vi "fx3u以太网通讯.vi"() -> ()   [LabVIEW 2017]
uses:
  C:/Users/Administrator/Desktop/LV2014_HslCommunication/LV2014_HslCommunication/HslCommunication.dll
  LV2014_HslCommunication/LV2014_HslCommunication/HslCommunication.dll
panel:
  out "Content 2":u32[](array[numeric])
  in  "布尔":bool
  out "IsSuccess 2":bool
  out "Content":i16
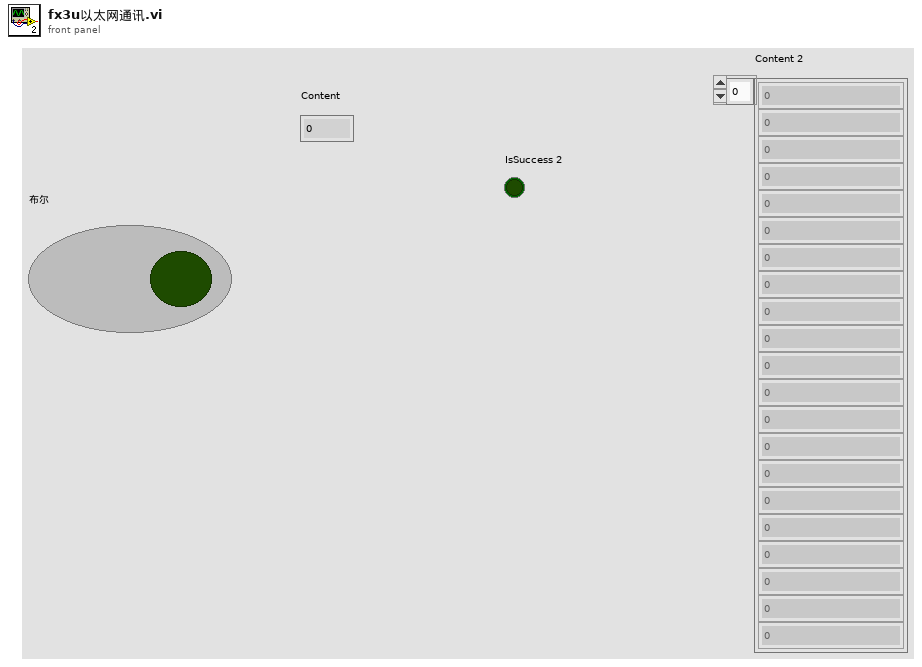
[diagram p1: front panel]
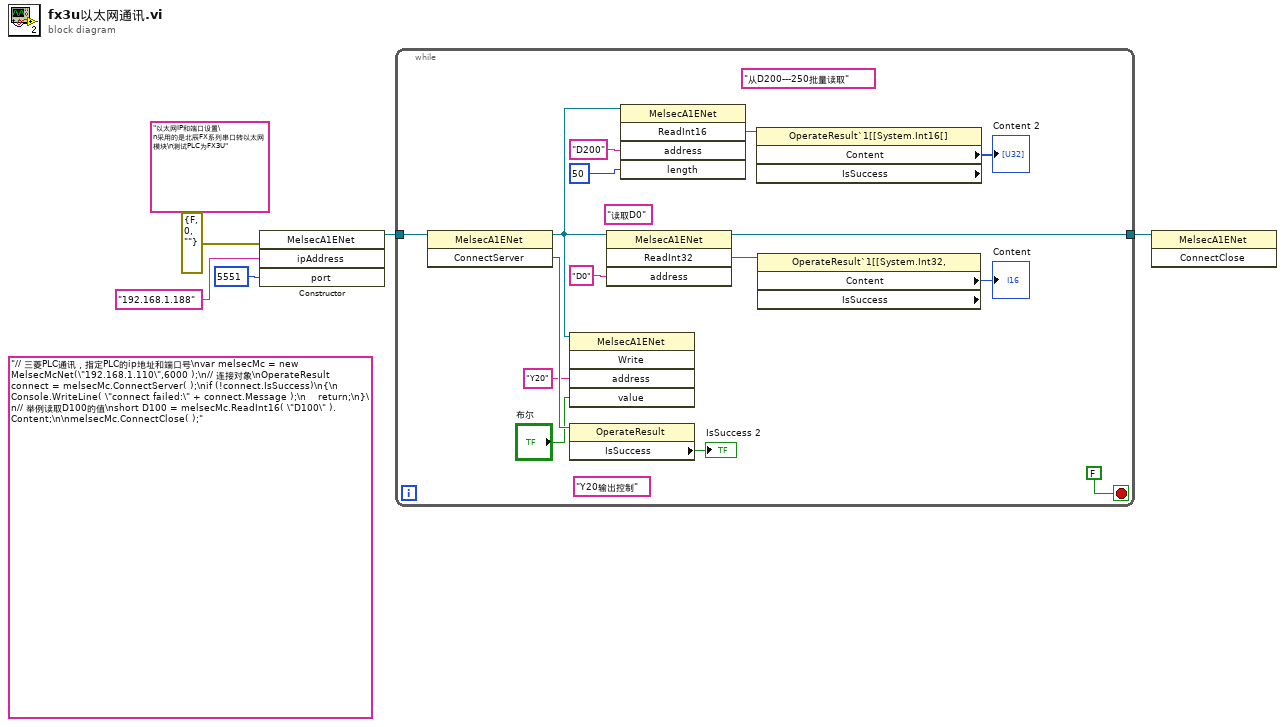
[diagram p0: block diagram]
diagram:
  (unwired) "以太网IP和端口设置\n采用的是北辰FX系列串口转以太网模块\n测试PLC为FX3U"
  (unwired) "// 三菱PLC通讯，指定PLC的ip地址和端口号\nvar melsecMc = new MelsecMcNet(\"192.168.1.110\",6000 );\n// 连接对象\nOperateResult connect = melsecMc.ConnectServer( );\nif (!connect.IsSuccess)\n{\n    Console.WriteLine( \"connect failed:\" + connect.Message );\n    return;\n}\n// 举例读取D100的值\nshort D100 = melsecMc.ReadInt16( \"D100\" ).Content;\n\nmelsecMc.ConnectClose( );"
  n1 = constructor class="MelsecA1ENet"(error in=errorcluster {"status"=FALSE, "code"=0, "source"=""} ("错误输入（无错误）"), "ipAddress"="192.168.1.188", "port"=5551) -> (reference out=w3:refnum<k24>)  [unwired: 2 in, 4 out]
  n2 = while {
    tunnel: [w16] -> w4
    tunnel: w3 -> [w14]
    stop <- FALSE stop-if-true
    (unwired) "读取D0"
    (unwired) "从D200---250批量读取"
    (unwired) "Y20输出控制"
    n3 = invoke class="MelsecA1ENet" method="ConnectServer"(reference=w14) -> (reference out=w10:refnum<k24>, "ConnectServer"=w13:refnum<k24>)  [unwired: 2 in, 1 out]
    n4 = invoke class="MelsecA1ENet" method="Write"(reference=w10, "address"="Y20", "value"="布尔") -> ()  [unwired: 2 in, 5 out]
    n5 = property class="OperateResult"(reference=w13) -> ("IsSuccess"=→"IsSuccess 2":bool)  [unwired: 1 in, 2 out]
    n6 = invoke class="MelsecA1ENet" method="ReadInt32"(reference=w10, "address"="D0") -> (reference out=w16:refnum<k24>, "ReadInt32"=w19:refnum<k24>)  [unwired: 2 in, 2 out]
    n7 = invoke class="MelsecA1ENet" method="ReadInt16"(reference=w10, "address"="D200", "length"=u16 50) -> ("ReadInt16"=w8:refnum<k24>)  [unwired: 2 in, 4 out]
    n8 = property class="OperateResult`1[[System.Int16[]" props=["Content", "IsSuccess"](reference=w8) -> ("Content"=→"Content 2":i16[])  [unwired: 1 in, 3 out]
    n9 = property class="OperateResult`1[[System.Int32, " props=["Content", "IsSuccess"](reference=w19) -> ("Content"=→"Content":i32)  [unwired: 1 in, 3 out]
  }
  n10 = invoke class="MelsecA1ENet" method="ConnectClose"(reference=w4) -> ()  [unwired: 2 in, 3 out]
